vi "controlAQuadBOutResolution.vi"(7 "Set":bool, 8 "error in":errorcluster, 9 "ABoutRes in":i32, 10 "axis in":u8, 11 "connection ID":i32) -> (0 "error out":errorcluster, 1 "ABoutRes out":i32, 2 "axis out":u8, 3 "connection ID":i32)   [LabVIEW 2016]
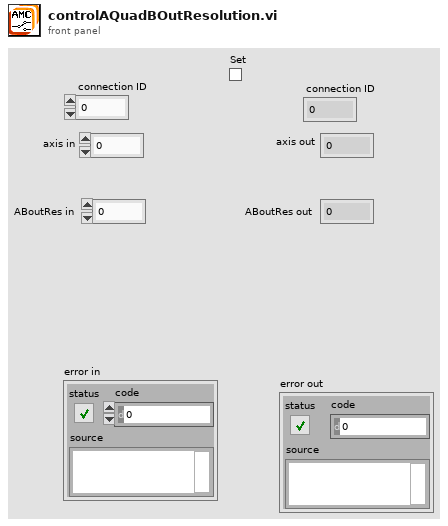
[diagram p1: front panel]
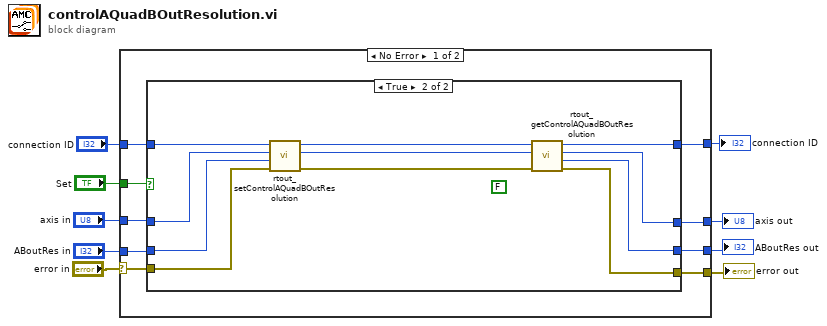
[diagram p0: block diagram]
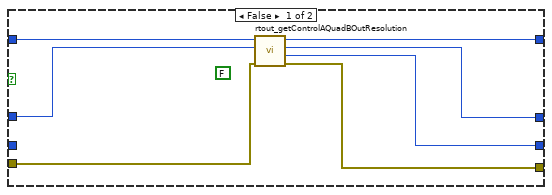
[diagram p2: hidden frame]
diagram:
  n1 = case shown="No Error" "error in" {
    selector: "error in" -> [w10 w39]
    tunnel: "axis in" -> [w16 w38]
    tunnel: [w11 w39] -> w8
    tunnel: [w13 w38] -> w7
    tunnel: "Set" -> [w17 _]
    tunnel: [w14 w37] -> w5
    tunnel: "connection ID" -> [w18 w37]
    tunnel: "ABoutRes in" -> [w15 w40]
    tunnel: [w12 w40] -> w2
    frame No Error {
      n2 = case shown="True" w17 {
        tunnel: [w24 w31] -> w14
        tunnel: w18 -> [w25 w36]
        tunnel: w16 -> [w21 w34]
        tunnel: [w20 w27] -> w13
        tunnel: [w19 w28] -> w12
        tunnel: [w22 w29] -> w11
        tunnel: w15 -> [_ w33]
        tunnel: w10 -> [w23 w35]
        frame False {
          (unwired) FALSE ("tempvalue")
          n3 = call "rtout_getControlAQuadBOutResolution.vi"("error in"=w23, "axis"=w21, "connection ID"=w25) -> ("error out"=w22:errorcluster, "resolution"=w19:i32, "axis_out"=w20:i32, "connection ID"=w24:i32)  [unwired: 5 in]
        }
        frame True {
          (unwired) FALSE ("tempvalue")
          n4 = call "rtout_setControlAQuadBOutResolution.vi"("error in"=w35, "resolution"=w33, "axis"=w34, "connection ID"=w36) -> ("error out"=w30:errorcluster, "axis_out"=w26:i32, "connection ID"=w32:i32)  [unwired: 5 in]
          n5 = call "rtout_getControlAQuadBOutResolution.vi"("error in"=w30, "axis"=w26, "connection ID"=w32) -> ("error out"=w29:errorcluster, "resolution"=w28:i32, "axis_out"=w27:i32, "connection ID"=w31:i32)  [unwired: 5 in]
        }
      }
    }
    frame Error {
    }
  }
  "error out" <- w8
  "axis out" <- w7
  "connection ID" <- w5
  "ABoutRes out" <- w2
